vi "visionglobal.vi"(8 "Set(T)/Get(F)":bool=TRUE, 11 "VisionAngle In":dbl format="%#_13g") -> (3 "VisionAngle Out":dbl format="%#_13g")   [LabVIEW 2017]
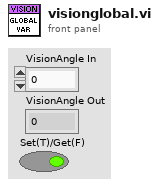
[diagram p1: front panel]
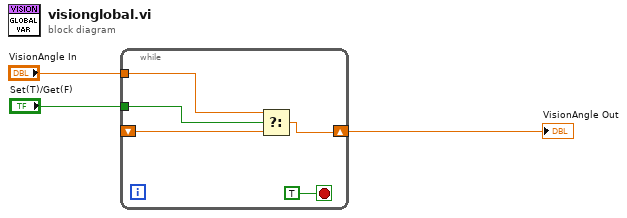
[diagram p0: block diagram]
diagram:
  n1 = while {
    shift-right: [w5] -> w2
    shift-left: _ -> [w6]
    tunnel: "Set(T)/Get(F)" -> [w7]
    tunnel: "VisionAngle In" -> [w4]
    stop <- TRUE stop-if-true
    n2 = Select(t=w4, s=w7, f=w6) -> (s? t:f=w5:dbl)
  }
  "VisionAngle Out" <- w2
